vi "Autodetect RTM.vi"(8 "error in (no error)":errorcluster, 11 "Node Ptr":u64 format="%.0x") -> (0 "error out":errorcluster)   [LabVIEW 2017, in "SLSC Switch System Explorer.lvlib"]
uses:
  SLSC Switch System Explorer.lvlib
  Scripting/VeriStand SLSC Scripting/VeriStand SLSC Scripting.lvlib
  Scripting/SLSC Switch Scripting.lvlib
panel:
  in  "Tag":string
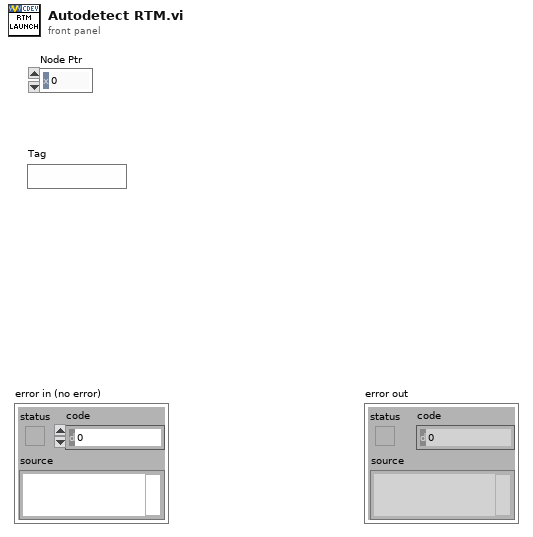
[diagram p1: front panel]
types:
  T1 = typedef "Custom Device API.lvlib/Custom Device Item Ref.ctl" = u64
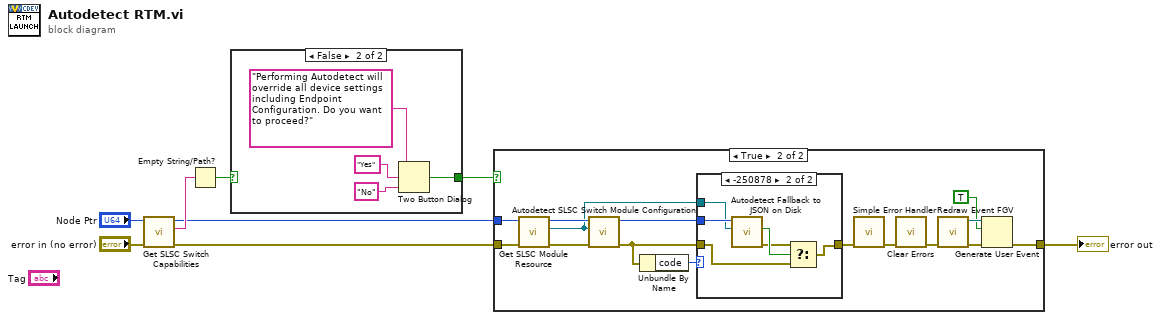
[diagram p0: block diagram]
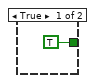
[diagram p4: hidden frame]
diagram:
  n1 = call "Get SLSC Switch Capabilities.vi"("error in (no error)"="error in (no error)", "SLSC Switch Custom Device Ref in"="Node Ptr") -> ("error out"=w1:errorcluster, "Capabilities"=w4:string, "SLSC Switch Custom Device Ref out"=w3:T1)  [unwired: 7 in]
  n2 = Empty String/Path?(string/path=w4) -> (empty?=w2:bool)
  n3 = case shown="False" w2 {
    tunnel: [TRUE ("T button?") w12] -> w7
    frame True {
    }
    frame False {
      n4 = Two Button Dialog(message="Performing Autodetect will override all device settings including Endpoint Configuration. Do you want to proceed?", 1:"No" ("F button name (\"Cancel\")"), 2:"Yes" ("T button name (\"OK\")")) -> (T button?=w12:bool)
    }
  }
  n5 = case shown="True" w7 {
    tunnel: w3 -> [_ w29]
    tunnel: w1 -> [w14 w28]
    tunnel: [w14 w22] -> w8
    frame False {
    }
    frame True {
      n6 = call "Get SLSC Module Resource.vi"("error in (no error)"=w28, "SLSC Module"=w29) -> ("error out"=w23:errorcluster, "SLSC Module Resource"=w16:refnum<k21>, "SLSC Module out"=w24:T1)  [unwired: 7 in]
      n7 = call "Autodetect SLSC Switch Module Configuration.vi"("error in"=w23, "SLSC Module"=w16, "SLSC Switch Custom Device Ref in"=w24) -> ("error out"=w19:errorcluster, "SLSC Switch Custom Device Ref out"=w15:T1)  [unwired: 7 in]
      n8 = Unbundle By Name(w19) -> ("code"=w18:i32)
      n9 = case shown="-250878" w18 {
        tunnel: w19 -> [w30 w33]
        tunnel: [w30 w31] -> w17
        tunnel: w16 -> [_ w35]
        tunnel: w15 -> [_ w36]
        frame Default {
        }
        frame -250878 {
          n10 = call "Autodetect Fallback to JSON on Disk.vi"("SLSC Module Resource"=w35, "SLSC Switch Custom Device Ref in"=w36) -> ("error out"=w32:errorcluster, "Fallback successful?"=w34:bool)  [unwired: 7 in, 1 out]
          n11 = Select(t=w32, s=w34, f=w33) -> (s? t:f=w31:errorcluster)
        }
      }
      n12 = call <vilib>:"Simple Error Handler.vi"("error in (no error)"=w17) -> ("error out"=w21:errorcluster)  [unwired: 4 in, 4 out]
      n13 = call <vilib>:"Clear Errors.vi"("error in (no error)"=w21) -> ("error out"=w20:errorcluster)  [unwired: 5 in, 1 out]
      n14 = call "Redraw Event FGV.vi"("error in (no error)"=w20) -> ("error out"=w27:errorcluster, "Redraw Event"=w26:refnum<user-event>)  [unwired: 9 in]
      n15 = Generate User Event(user event=w26, event data cluster=TRUE ("event data"), error in=w27) -> (error out=w22:errorcluster)  [unwired: 1 in, 1 out]
    }
  }
  "error out" <- w8
